vi "User32dllAPI.ShowWindow.vi"(8 "error in (no error)":errorcluster, 10 "Cmd":T1=5 items=["HIDE"=0, "MAXIMIZE"=3, "SHOW"=5, "MINIMIZE"=6], 11 "hWnd":i32) -> (0 "error out":errorcluster, 3 "hWnd out":i32)   [LabVIEW 2010]
uses:
  User32dllAPI.ShowWindow.Cmd.ctl
  user32.dll
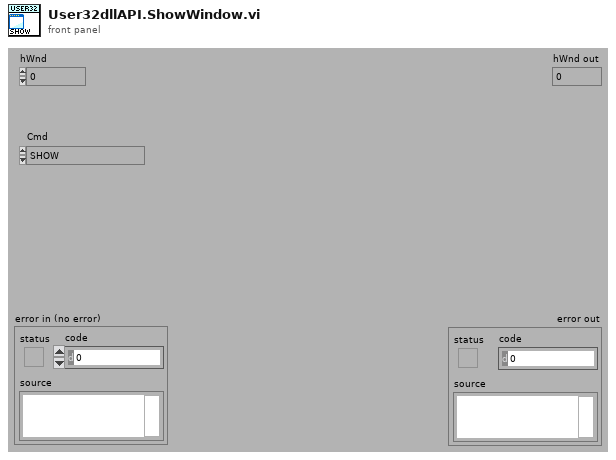
[diagram p1: front panel]
types:
  T1 = typedef "User32dllAPI.ShowWindow.Cmd.ctl" = i32
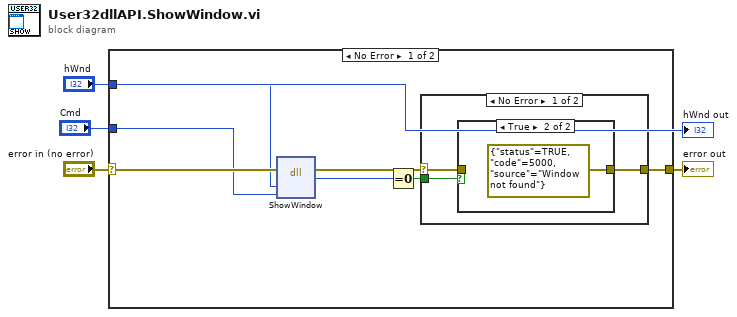
[diagram p0: block diagram]
diagram:
  n1 = case shown="No Error" "error in (no error)" {
    selector: "error in (no error)" -> [w10 w18]
    tunnel: [w8 w18] -> w3
    tunnel: "hWnd" -> [w7 _]
    tunnel: "Cmd" -> [w5 _]
    frame No Error {
      n2 = dll-call lib="USER32.DLL" fn="ShowWindow"(error in=w10, "hWnd"=w7, "nCmdShow"=w5) -> (error out=w9:errorcluster, "result"=w6:i32)  [unwired: 4 in, 1 out]
      n3 = Equal To 0?(x=w6) -> (x = 0?=w11:bool)
      n4 = case shown="No Error" w9 {
        selector: w9 -> [w12 w17]
        tunnel: w11 -> [w14 _]
        tunnel: [w13 w17] -> w8
        frame No Error {
          n5 = case shown="True" w14 {
            tunnel: [w15 errorcluster {"status"=TRUE, "code"=5000, "source"="Window not found"} ("error out")] -> w13
            tunnel: w12 -> [w15 _]
            frame False {
            }
            frame True {
            }
          }
        }
        frame Error {
        }
      }
    }
    frame Error {
    }
  }
  "error out" <- w3
  "hWnd out" <- "hWnd"
